vi "file kosong.vi"   [LabVIEW 2016, in "Test2.lvrbt"]
uses:
  Test2.lvrbt
  <vilib>/NXT/Block Support/NXT_InputPort.ctl
  <vilib>/NXT/Hardware/Plugins/Tetrix DC Motor/TetrixDCMotorAddress.ctl
  <vilib>/NXT/NXTIO Xnodes/NXTIONodeSubVIs/TETRIX IO Move DC Motors.vi
  <vilib>/NXT/Dual Mode Library/Waits/Wait_EV3_Ultrasonic_Centimeter_Closer.vi
  <vilib>/NXT/NXTIO Xnodes/NXTIONodeSubVIs/TETRIX IO Stop DC Motors.vi
  <vilib>/NXT/Dual Mode Library/Waits/Wait_Num.vi
  <vilib>/NXT/Dual Mode Library/Waits/Wait_EV3_Ultrasonic_Centimeters_Further.vi
  <vilib>/NXT/Subs/LVHSConnector.ctl
  <vilib>/NXT/NXTIO Xnodes/AddressXNode/NXTIOAddress.xnode
  <vilib>/NXT/NXTIO Xnodes/NXTIOXNode/NXTIO.xnode
  <vilib>/NXT/LegoClasses/BrickReference/BrickReference.lvclass
types:
  T1 = typedef "NXT_InputPort.ctl" = u32
  T2 = typedef "TetrixDCMotorAddress.ctl" = i32
  T3 = typedef "LVHSConnector.ctl" = refnum<class "BrickReference.lvclass">
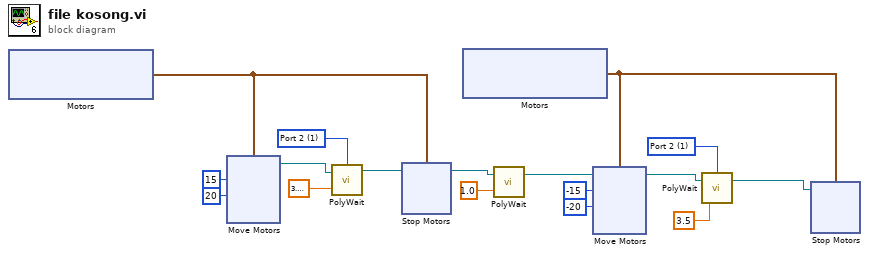
[diagram p0: block diagram]
diagram:
  w3 = T1 1 items=["Port 1", "Port 2", "Port 3", "Port 4"] ("Port (Port 1)")
  w13 = T1 1 items=["Port 1", "Port 2", "Port 3", "Port 4"] ("Port (Port 1)")
  n1 = xnode "Motors"() -> ("Motor"=w11:cluster{"TetrixDCMotor":T2, "TetrixDCMotor":T2})
  n2 = xnode "Move Motors"("Power/Speed 2"=i8 20, "Power/Speed 1"=i8 15, "Motors"=w11) -> ("NXT/EV3"=w15:T3)  [unwired: 1 in]
  n3 = call-poly <vilib>:"PolyWait.vi"("Centimeters (40)"=sgl 3.1 ("Time (1 sec)"), "NXT/EV3"=w15, "Port (Port 1)"=w13) -> ("NXT/EV3"=w12:T3)  [unwired: 1 in]
  n4 = xnode "Stop Motors"("Motors"=w11, "NXT/EV3"=w12) -> ("NXT/EV3"=w10:T3)
  n5 = xnode "Motors"() -> ("Motor"=w1:cluster{"TetrixDCMotor":T2, "TetrixDCMotor":T2})
  n6 = call-poly <vilib>:"PolyWait.vi"("Time (1 sec)"=sgl 1.0, "NXT/EV3"=w10) -> ("NXT/EV3"=w8:T3)  [unwired: 2 in]
  n7 = xnode "Move Motors"("Power/Speed 2"=i8 -20, "Power/Speed 1"=i8 -15, "Motors"=w1, "NXT/EV3"=w8) -> ("NXT/EV3"=w5:T3)
  n8 = call-poly <vilib>:"PolyWait.vi"("Centimeters (50)"=sgl 3.5, "NXT/EV3"=w5, "Port (Port 1)"=w3) -> ("NXT/EV3"=w2:T3)  [unwired: 1 in]
  n9 = xnode "Stop Motors"("Motors"=w1, "NXT/EV3"=w2) -> ()  [unwired: 1 out]
